vi "LIA-PollData.vi"(0 "Address":string="DEV", 1 "stop":bool) -> (17 "theta (deg)":dbl[](array[numeric]), 20 "Selected Device":string, 21 "Demod R (V)":dbl format="%_4p", 22 "Demod Phi (rad)":dbl format="%.3p", 23 "Spectral Density\nVrms/sqrt(Hz)":dbl=1.331104953906021e-08 format="%0.2p", 25 "Demod Sample Out":T3 {"Aux In 1 (V)" format="%#_5p"; "Aux In 0 (V)" format="%#_5p"; "X (Vrms)" format="%#_5p"; "Y (Vrms)" format="%#_5p"; "Osc Phase (rad)" format="%#.3g"}, 26 "DIO Out":T2, 27 "AuxIn Out":T1)   [LabVIEW 2016]
doc: "Control a Zurich instrument device via the LabOne Labview API. \nRequirements: Zurich Instruments MFLI, HF2 or UHFLI \nThis example polls data from the instrument.\n\n© Zurich Instruments AG, www.zhinst.com"
uses:
  <instrlib>/Zurich Instruments LabOne/Public/Data/ziTypeDemodSampleEx.ctl
  <instrlib>/Zurich Instruments LabOne/Public/Data/ziTypeAuxInSample.ctl
  <instrlib>/Zurich Instruments LabOne/Public/Configure/ziSetValueDoubleArray.vi
  <instrlib>/Zurich Instruments LabOne/Public/Configure/ziGetValueDouble.vi
  <instrlib>/Zurich Instruments LabOne/Public/Data/ziGetEventAuxInSample.vi
  <instrlib>/Zurich Instruments LabOne/Public/Data/ziGetEventDemodSample.vi
  <instrlib>/Zurich Instruments LabOne/Public/Data/ziGetEventDIOSample.vi
  <instrlib>/Zurich Instruments LabOne/Zurich Instruments LabOne.lvlib
panel:
  out "Error Out":errorcluster
  in  "Edge":u16(ring)=1 items=["Off", "Rising Edge", "Falling Edge", "Both Edges"]
  in  "DIO Channel":u16(ring) items=["Continous"=0, "DIO 0 / Tigger 3"=1, "DIO 1 / Tigger 4"=4, "DIO 0|1 / Tigger 3|4"=5]
  out "Demod sample":dbl[](graph)
  out "DIO":u32[](graph)
  out "AUX Input":dbl[](graph)
  # "ziExample-PollData.vi\nRequirements: HF2, UHFLI or MFLI\nsee block diagram for VI description"
  # "Tested Instruments:\n- MFLI\n- HF2LI\n- UHFLI"
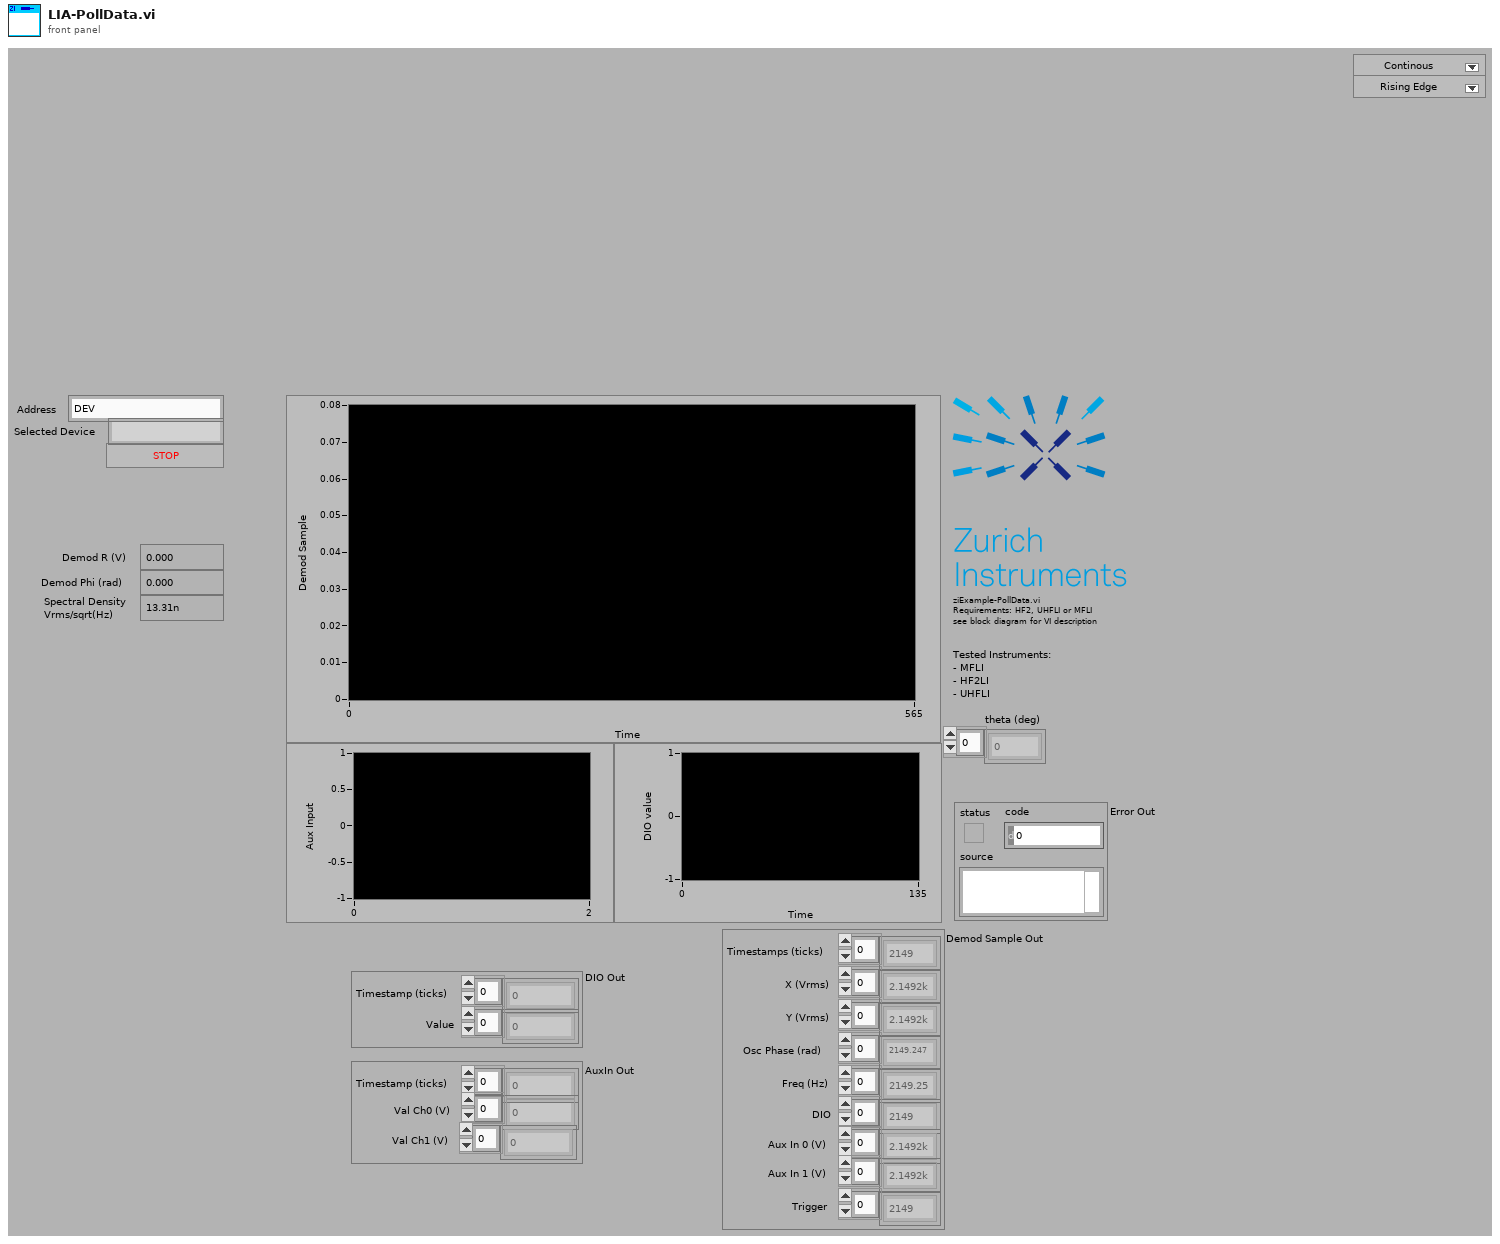
[diagram p1: front panel]
types:
  T1 = typedef "Zurich Instruments LabOne.lvlib/ziTypeAuxInSample.ctl" = cluster{"Timestamp (ticks)":u64[], "Val Ch0 (V)":dbl[], "Val Ch1 (V)":dbl[]}
  T2 = cluster{"Timestamp (ticks)":u64[], "Value":u32[]}
  T3 = typedef "Zurich Instruments LabOne.lvlib/ziTypeDemodSampleEx.ctl" = cluster{"Timestamps (ticks)":u64[], "X (Vrms)":dbl[], "Y (Vrms)":dbl[], "Osc Phase (rad)":dbl[], "Freq (Hz)":dbl[], "DIO":u32[], "Aux In 0 (V)":dbl[], "Aux In 1 (V)":dbl[], "Trigger":u32[]}
  T4 = cluster{"Path":string, "Value":dbl, "comment":string}[]
  T5 = typedef "Zurich Instruments LabOne.lvlib/ziTypeHandle.ctl" = cluster{"handleValid":bool, "Conn":u64, "Path Prefix":string, "Handle":u64, "Connected":bool, "Clockbase(s)":dbl}
  T6 = typedef "Zurich Instruments LabOne.lvlib/ziTypePollType.ctl" = enum16{"NONE", "DOUBLE_DATA", "INTEGER_DATA", "DEMOD_SAMPLE", "SCOPE_WAVE_HF2", "AUXIN_SAMPLE", "DIO_SAMPLE", "BYTE_ARRAY", "PWA_WAVE", "9", "10", "11", "12", "13", "14", "15", "TREE_CHANGE_DEPRI", "17", "ERROR", "19", "20", "21", "22", "23", "24", "25", "26", "27", "28", "29", "30", "31", "DOUBLE_DATA_TS", "INTEGER_DATA_TS", "34", "SCOPE_WAVE", "SCOPE_WAVE_EX", "37", "BYTE_ARRAY_TS", "39", "40", "41", "42", "43", "44", "45", "CNT_DATA", "47", "TREE_CHANGE", "49", "50", "51", "52", "53", "54", "55", "56", "57", "58", "59", "60", "61", "62", "63", "SWEEPER_DATA", "SPECTRUM_DATA", "ADVISOR_DATA", "VECTOR_DATA", "IMP_DATA"}
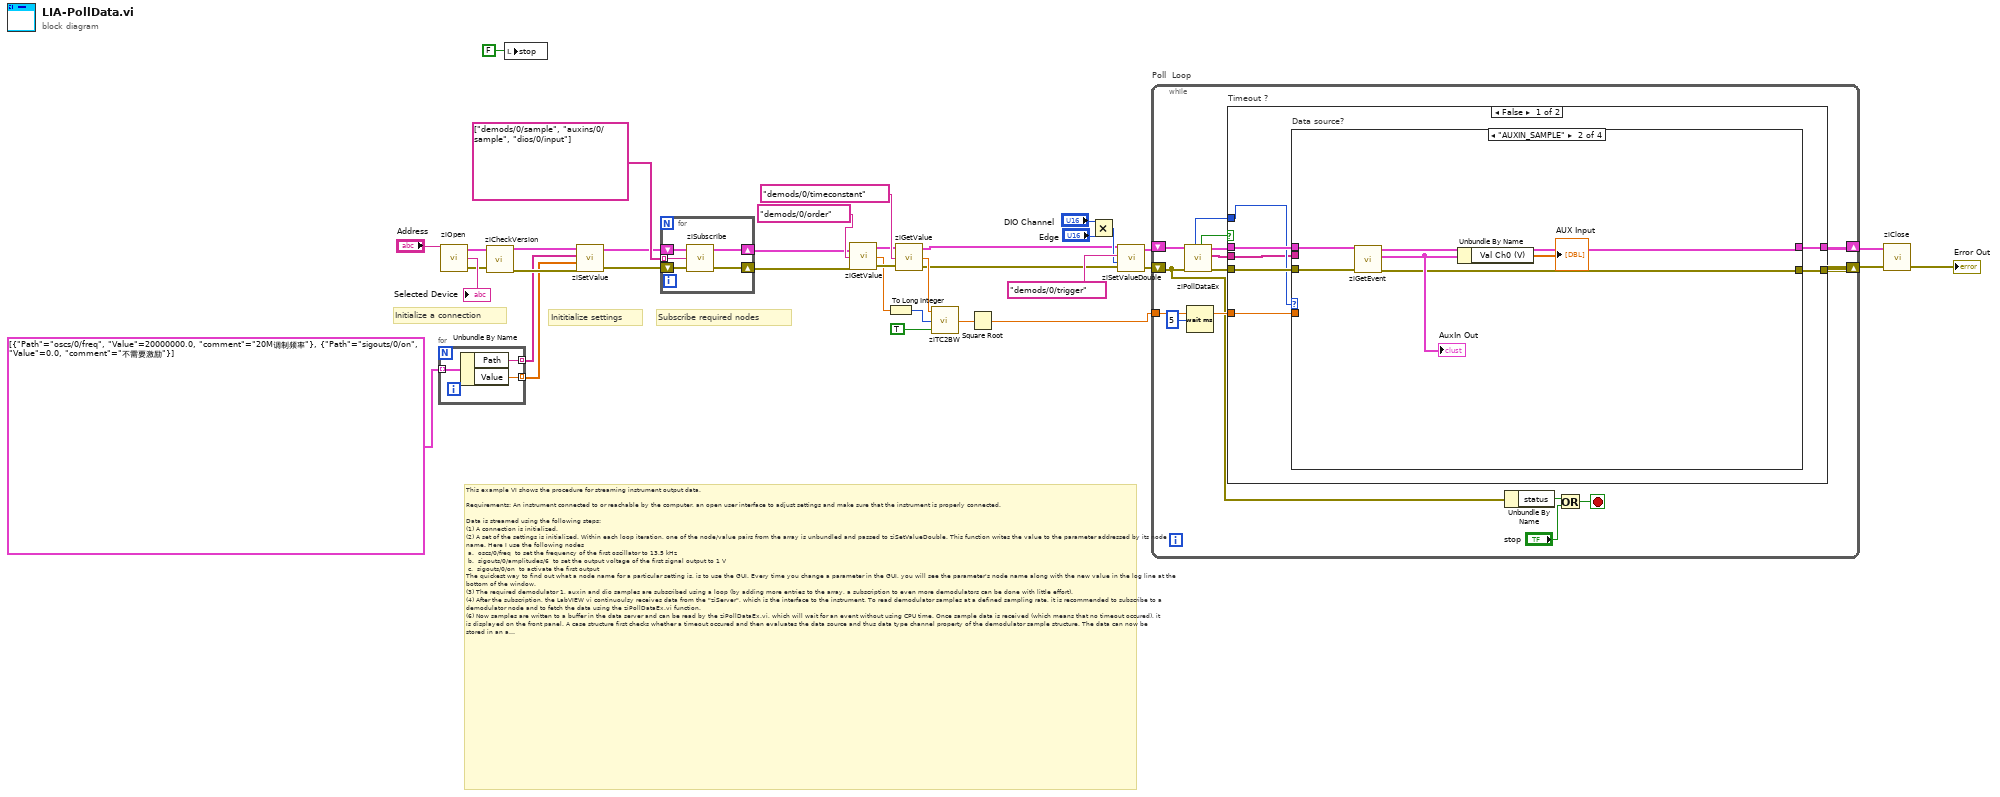
[diagram p0: block diagram]
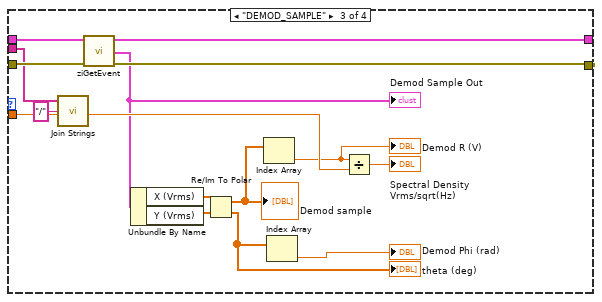
[diagram p3: hidden frame]
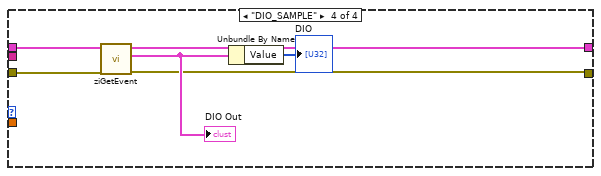
[diagram p4: hidden frame]
diagram:
  # "Inititialize settings"
  # "Initialize a connection"
  # "Subscribe required nodes"
  # "This example VI shows the procedure for streaming instrument output data.\n\nRequirements: An instrument connected to or reachable by the computer, an open user interface to adjust settings and make sure that the instrument is properly connected. \n\nData is streamed using the following steps:\n(1) A connection is initialized.\n(2) A set of the settings is initialized. Within each loop iteration, one of the node/value pairs from the array is unbundled and passed to ziSetValueDouble. This function writes the value to the parameter addressed by its node name. Here I use the following nodes\n a. \toscs/0/freq \tto set the frequency of the first oscillator to 13.5 kHz\n b. \tsigouts/0/amplitudes/6 \tto set the output voltage of the first signal output to 1 V\n c. \tsigouts/0/on \tto activate the first output\nThe quickest way to find out what a node name for a particular setting is, is to use the GUI. Every time you change a parameter in the GUI, you will see the parameter's node name along with the new value in the log line at the bottom of the window. \n(3) The required demodulator 1, auxin and dio samples are subscribed using a loop (by adding more entries to the array, a subscription to even more demodulators can be done with little effort).\n(4) After the subscription, the LabVIEW vi continuoulsy receives data from the \"ziServer\", which is the interface to the instrument. To read demodulator samples at a defined sampling rate, it is recommended to subscribe to a demodulator node and to fetch the data using the ziPollDataEx.vi function. \n(6) Now samples are written to a buffer in the data server and can be read by the ziPollDataEx.vi, which will wait for an event without using CPU time. Once sample data is received (which means that no timeout occured), it is displayed on the front panel. A case structure first checks whether a timeout occured and then evaluates the data source and thus data type channel property of the demodulator sample structure. The data can now be stored in an array or a queue or be shown in a waveform chart. \n(7) Finally, the connection is closed. \n \n© Zurich Instruments AG, 2016, www.zhinst.com"
  n1 = for {
    tunnel: T4 [{"Path"="oscs/0/freq", "Value"=20000000.0, "comment"="20M调制频率"}, {"Path"="sigouts/0/on", "Value"=0.0, "comment"="不需要激励"}] -> [w39] mode=indexing
    tunnel: [w38] -> w2 mode=indexing
    tunnel: [w37] -> w1 mode=indexing
    n2 = Unbundle By Name(w39) -> ("Path"=w38:string, "Value"=w37:dbl)
  }
  n3 = call <instrlib>:"ziOpen.vi"("Address"="Address") -> ("Error Out"=w7:errorcluster, "Selected Device"=→"Selected Device":string, "HandleOut"=w8:T5)  [unwired: 1 in, 2 out]
  n4 = call <instrlib>:"ziCheckVersion.vi"("Handle In"=w8, "Error In"=w7) -> ("Handle Out"=w5:T5, "Error Out"=w6:errorcluster)  [unwired: 11 in, 1 out]
  n5 = local write "stop"(FALSE ("stop")) -> ()
  n6 = call-poly <instrlib>:"ziSetValue.vi"("Error In"=w6, "Values"=w1, "Paths"=w2, "Handle In"=w5) -> ("Error Out"=w33:errorcluster, "Handle Out"=w34:T5)  [unwired: 1 in]
  n7 = for {
    shift-right: [w44] -> w21
    shift-left: w34 -> [w42]
    shift-right: [w43] -> w20
    shift-left: w33 -> [w41]
    tunnel: string[] ["demods/0/sample", "auxins/0/sample", "dios/0/input"] -> [w40] mode=indexing
    n8 = call <instrlib>:"ziSubscribe.vi"("error in"=w41, "Path ()"=w40, "Handle In"=w42) -> ("error out"=w43:errorcluster, "Handle Out"=w44:T5)  [unwired: 1 in]
  }
  n9 = call-poly <instrlib>:"ziGetValue.vi"("error in"=w20, "Path"="demods/0/order", "Handle in"=w21) -> ("error out"=w27:errorcluster, "Value"=w26:dbl, "Handle out"=w28:T5)
  n10 = To Long Integer(number=w26) -> (32bit integer=w25:i32)
  n11 = call-poly <instrlib>:"ziGetValue.vi"("error in"=w27, "Path"="demods/0/timeconstant", "Handle in"=w28) -> ("error out"=w10:errorcluster, "Value"=w24:dbl, "Handle out"=w11:T5)
  n12 = call <instrlib>:"ziTC2BW.vi"("Eq BW (F)"=TRUE ("Eq BW"), "Order (1)"=w25, "TC (s)"=w24) -> ("BW (Hz)"=w23:dbl)
  n13 = Square Root(x=w23) -> (sqrt(x)=w19:dbl)
  n14 = Multiply(x="DIO Channel", y="Edge") -> (x*y=w16:u16)
  n15 = call <instrlib>:"ziSetValueDouble.vi"("Error In"=w10, "Value"=w16, "Path"="demods/0/trigger", "Handle In"=w11) -> ("Error Out"=w13:errorcluster, "Handle Out"=w12:T5)  [unwired: 1 in]
  n16 = while "Poll  Loop" {
    shift-right: [w58] -> w36
    shift-left: w12 -> [w50]
    shift-right: [w54] -> w18
    shift-left: w13 -> [w47]
    tunnel: w19 -> [w52]
    stop <- w45 stop-if-true
    n17 = call <instrlib>:"ziPollDataEx.vi"("error in"=w47, "Handle In"=w50) -> ("error out"=w55:errorcluster, "PathArray"=w49:string[], "Handle Out"=w57:T5, "Timed Out"=w56:bool, "ziValueType"=w53:T6)  [unwired: 2 in, 3 out]
    n18 = Wait (ms)(milliseconds to wait=u32 5) -> ()  [unwired: 1 out]
    n19 = case "Timeout ?" shown="False" w56 {
      tunnel: w57 -> [w65 w96]
      tunnel: [w64 w96] -> w58
      tunnel: w55 -> [w63 w95]
      tunnel: [w62 w95] -> w54
      tunnel: w53 -> [w60 _]
      tunnel: w52 -> [w61 _]
      tunnel: w49 -> [w59 _]
      frame False {
        n20 = case "Data source?" shown="\"AUXIN_SAMPLE\"" w60 {
          tunnel: w65 -> [w67 w73 w88 w94]
          tunnel: [w67 w71 w87 w93] -> w64
          tunnel: w63 -> [w66 w70 w86 w91]
          tunnel: [w66 w69 w85 w90] -> w62
          tunnel: w61 -> [_ _ w84 _]
          tunnel: w59 -> [_ _ w75 _]
          frame Default {
          }
          frame "AUXIN_SAMPLE" {
            n21 = call-poly <instrlib>:"ziGetEvent.vi"("Error In"=w70, "Handle In"=w73) -> ("Error Out"=w69:errorcluster, "AuxIn Out"=w72:T1, "Handle Out"=w71:T5)  [unwired: 7 in]
            "AuxIn Out" <- w72
            n22 = Unbundle By Name(w72) -> ("Val Ch0 (V)"=→"AUX Input":dbl[])
          }
          frame "DEMOD_SAMPLE" {
            n23 = call <vilib>:"Join Strings.vi"("Separator (,)"="/", "Strings In"=w75) -> ()  [unwired: 1 in, 1 out]
            n24 = call-poly <instrlib>:"ziGetEvent.vi"("Error In"=w86, "Handle In"=w88) -> ("Error Out"=w85:errorcluster, "Demod Sample Out"=w81:T3, "Handle Out"=w87:T5)  [unwired: 7 in]
            "Demod Sample Out" <- w81
            n25 = Unbundle By Name(w81) -> ("X (Vrms)"=w83:dbl[], "Y (Vrms)"=w82:dbl[])
            n26 = Re/Im To Polar(2:w82, 3:w83) -> (0:w78:dbl[], 1:w79:dbl[])
            "Demod sample" <- w79
            "theta (deg)" <- w78
            n27 = Index Array(array=w79) -> (element=w76:dbl)  [unwired: 1 in]
            "Demod R (V)" <- w76
            n28 = Index Array(array=w78) -> (element=→"Demod Phi (rad)":dbl)  [unwired: 1 in]
            n29 = Divide(x=w76, y=w84) -> (x/y=→"Spectral Density\nVrms/sqrt(Hz)":dbl)
          }
          frame "DIO_SAMPLE" {
            n30 = call-poly <instrlib>:"ziGetEvent.vi"("Error In"=w91, "Handle In"=w94) -> ("Error Out"=w90:errorcluster, "DIO Out"=w92:T2, "Handle Out"=w93:T5)  [unwired: 7 in]
            "DIO Out" <- w92
            n31 = Unbundle By Name(w92) -> ("Value"=→"DIO":u32[])
          }
        }
      }
      frame True {
        # "Timeout, no action."
      }
    }
    n32 = Unbundle By Name(w47) -> ("status"=w48:bool)
    n33 = Or(x=w48, y="stop") -> (x .or. y?=w45:bool)
  }
  n34 = call <instrlib>:"ziClose.vi"("Error In"=w18, "Handle In"=w36) -> ("Error Out"=→"Error Out":errorcluster)  [unwired: 3 out]
